vi "Hankel Matrix (DBL).vi"(10 "Input Vector2":dbl[](array[numeric]), 11 "Input Vector1":dbl[](array[numeric])) -> (0 "error":i32, 3 "Hankel Matrix":T1)   [LabVIEW 2020, in "NI_AALPro.lvlib"]
uses:
  NI_AALPro.lvlib
  RealMatrix.ctl
  NI_Matrix.lvlib
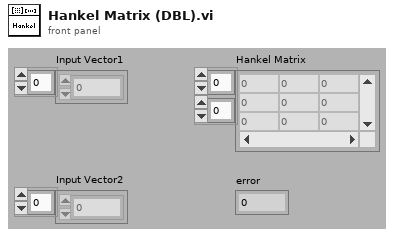
[diagram p1: front panel]
types:
  T1 = typedef "NI_Matrix.lvlib/RealMatrix.ctl" = dbl[][]
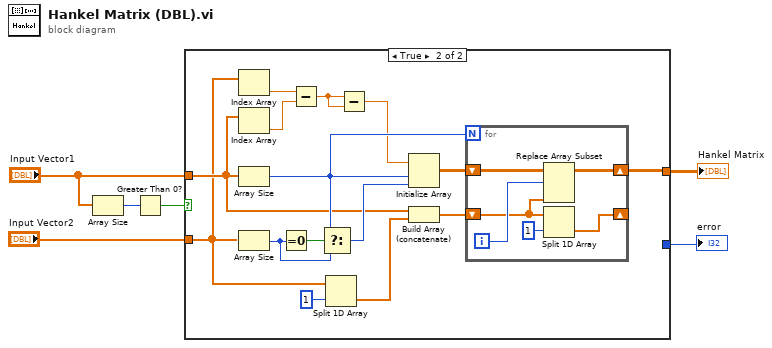
[diagram p0: block diagram]
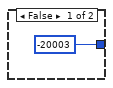
[diagram p2: hidden frame]
diagram:
  n1 = Array Size(array="Input Vector1") -> (size(s)=w4:i32)
  n2 = Greater Than 0?(x=w4) -> (x > 0?=w1:bool)
  n3 = case shown="True" w1 {
    tunnel: "Input Vector1" -> [_ w10]
    tunnel: "Input Vector2" -> [_ w9]
    tunnel: [_ w8] -> w6
    tunnel: [-20003 _] -> w3
    frame False {
    }
    frame True {
      n4 = Index Array(array=w9) -> (element=w13:dbl)  [unwired: 1 in]
      n5 = Index Array(array=w10) -> (element=w14:dbl)  [unwired: 1 in]
      n6 = Array Size(array=w10) -> (size(s)=w17:i32)
      n7 = Array Size(array=w9) -> (size(s)=w15:i32)
      n8 = Equal To 0?(x=w15) -> (x = 0?=w18:bool)
      n9 = Subtract(x=w13, y=w14) -> (x-y=w12:dbl)
      n10 = Select(t=w17, s=w18, f=w15) -> (s? t:f=w16:i32)
      n11 = Split 1D Array(array=w9, index=1) -> (second subarray=w20:dbl[])  [unwired: 1 out]
      n12 = Subtract(x=w12, y=w12) -> (x-y=w11:dbl)
      n13 = Initialize Array(w11, w17, w16) -> (w21:dbl[][])
      n14 = Build Array (concatenate)(w10, w20) -> (w22:dbl[])
      n15 = for {
        N: w17 -> [_]
        shift-right: [w23] -> _
        shift-left: w22 -> [w24]
        shift-right: [w27] -> w8
        shift-left: w21 -> [w28]
        i -> [w26]
        n16 = Replace Array Subset(array=w28, new element=w24, index (row)=w26) -> (w27:dbl[][])  [unwired: 1 in]
        n17 = Split 1D Array(array=w24, index=1) -> (second subarray=w23:dbl[])  [unwired: 1 out]
      }
    }
  }
  "Hankel Matrix" <- w6
  "error" <- w3
